vi "solar_gbl Read Config (Override).vi"(8 "error in (no error)":errorcluster, 9 "Default Targets (name,vi)":string[][](array[string]), 10 "Name in":string, 11 "SOLAR in":T1) -> (0 "error out":errorcluster, 1 "Targets (name,vi)":string[][](array[string]), 2 "Name out":string, 3 "SOLAR out":T1)   [LabVIEW 2018]
doc: "This loads the application setup override keys in the solar.ini configuration file. SOLAR uses the default application settings, to override add the key to override in the 'AppSetups' section.\nExample:\n[solar]\nAppSetups = \"Board,Box\"\nTitle = \"My Default App\"\n\n[Board]\nTitle = \"My Board App\""
uses:
  solar_ctl SOLAR Global.ctl
  solar_ctl Target Global.ctl
  voyager/solar_voy_ctl Voyager Refnum.ctl
  qtimer/solar_qtimer_ctl Refnum.ctl
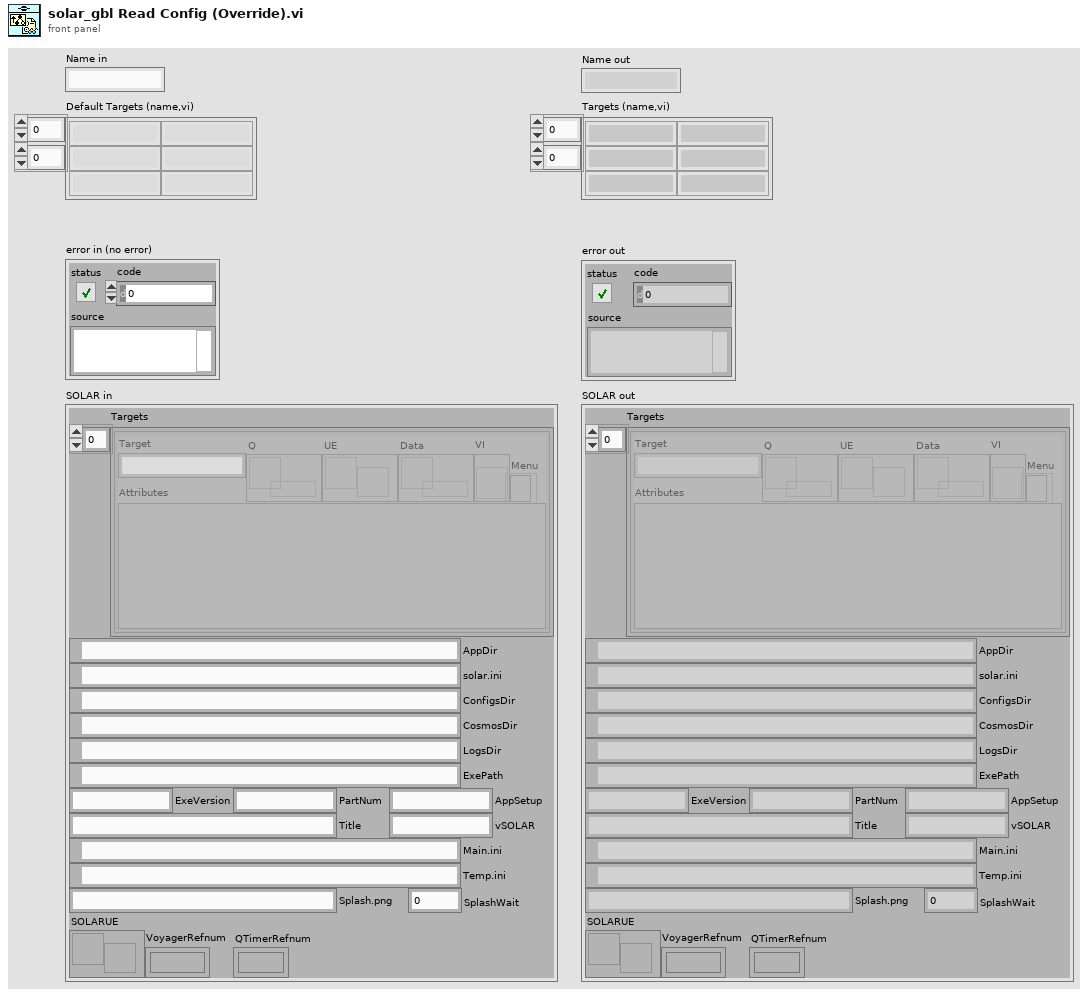
[diagram p1: front panel]
types:
  T1 = typedef "solar_ctl SOLAR Global.ctl" = cluster{"Targets":T2[], "AppDir":path, "solar.ini":path, "ConfigsDir":path, "CosmosDir":path, "LogsDir":path, "ExePath":path, "ExeVersion":string, "PartNum":string, "AppSetup":string, "Title":string, "Main.ini":path, "Temp.ini":path, "vSOLAR":string, "Splash.png":string, "SplashWait":i32, "SOLARUE":refnum<user-event>, "VoyagerRefnum":T3, "QTimerRefnum":T4}
  T2 = typedef "solar_ctl Target Global.ctl" = cluster{"Target":string, "Q":refnum<queue>, "UE":refnum<user-event>, "VI":refnum<vi>, "Menu":refnum<k9>, "Data":refnum<data-value>, "Attributes":variant}
  T3 = typedef "solar_voy_ctl Voyager Refnum.ctl" = refnum<k1>
  T4 = typedef "solar_qtimer_ctl Refnum.ctl" = refnum<k1>
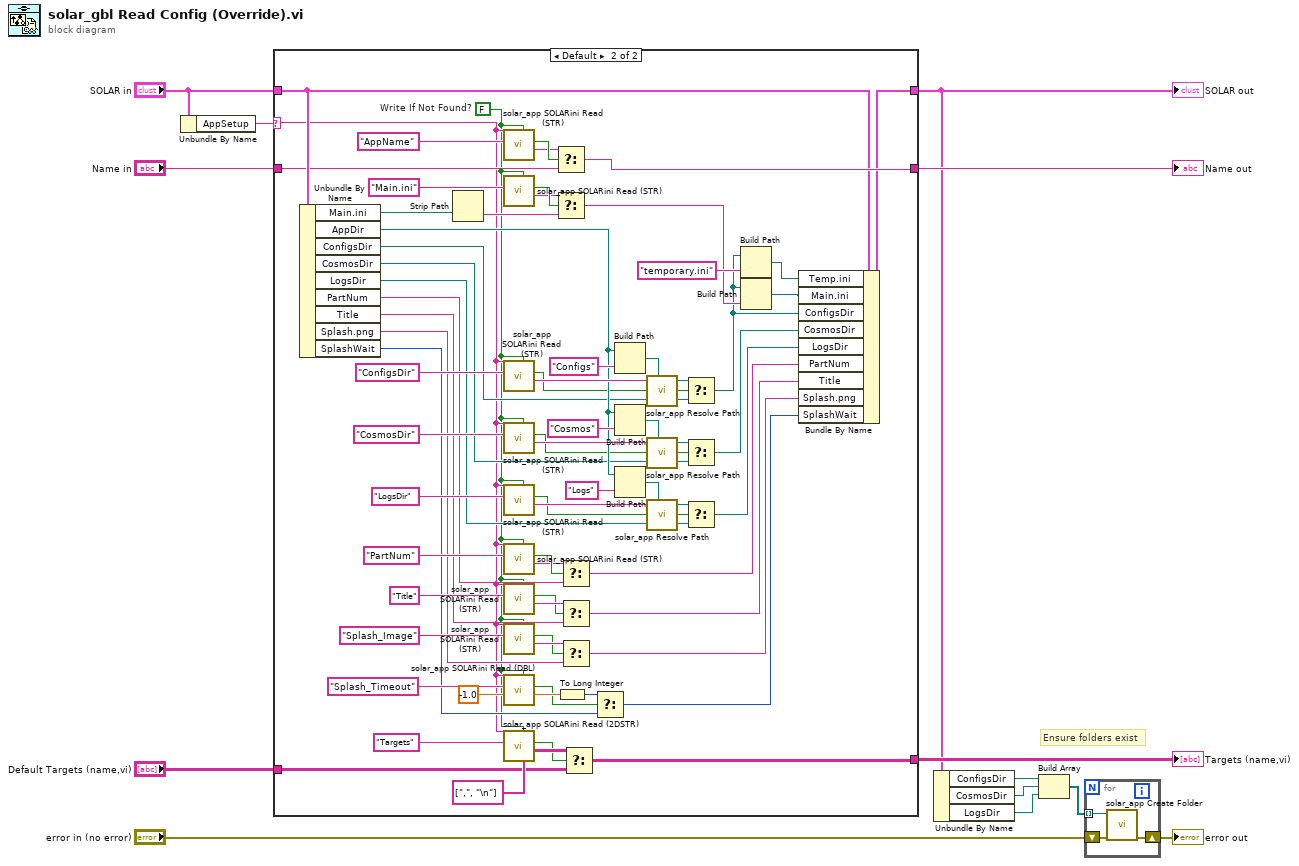
[diagram p0: block diagram]
diagram:
  # "Ensure folders exist"
  n1 = Unbundle By Name("SOLAR in") -> ("AppSetup"=w9:string)
  n2 = case shown="Default" w9 {
    selector: w9 -> [_ w18]
    tunnel: "Name in" -> [w15 w60]
    tunnel: [w15 w75] -> w12
    tunnel: [w16 w64] -> w1
    tunnel: [w14 w23] -> w11
    tunnel: "SOLAR in" -> [w16 w63]
    tunnel: "Default Targets (name,vi)" -> [w14 w24]
    frame "" {
      # "Use default configuration settings"
    }
    frame Default {
      w17 = FALSE  # Write If Not Found?
      n3 = Unbundle By Name(w63) -> ("Main.ini"=w58:path, "AppDir"=w53:path, "ConfigsDir"=w49:path, "CosmosDir"=w46:path, "LogsDir"=w40:path, "PartNum"=w37:string, "Title"=w33:string, "Splash.png"=w22:string, "SplashWait"=w20:i32)
      n4 = Strip Path(path=w58) -> (name=w57:string)  [unwired: 1 out]
      n5 = call "solar_app SOLARini Read (STR).vi"("Write If Not Found? (T)"=w17, "Section (\"\"=solar)"=w18, "Key"="AppName") -> ("Value (STR) out"=w61:string, "Found?"=w62:bool)  [unwired: 7 in]
      n6 = call "solar_app SOLARini Read (STR).vi"("Write If Not Found? (T)"=w17, "Key"="Main.ini") -> ("Value (STR) out"=w56:string, "Found?"=w59:bool)  [unwired: 8 in]
      n7 = call "solar_app SOLARini Read (STR).vi"("Write If Not Found? (T)"=w17, "Section (\"\"=solar)"=w18, "Key"="ConfigsDir") -> ("Value (STR) out"=w76:string, "Found?"=w51:bool)  [unwired: 7 in]
      n8 = call "solar_app SOLARini Read (STR).vi"("Write If Not Found? (T)"=w17, "Section (\"\"=solar)"=w18, "Key"="CosmosDir") -> ("Value (STR) out"=w78:string, "Found?"=w47:bool)  [unwired: 7 in]
      n9 = call "solar_app SOLARini Read (STR).vi"("Write If Not Found? (T)"=w17, "Section (\"\"=solar)"=w18, "Key"="LogsDir") -> ("Value (STR) out"=w81:string, "Found?"=w41:bool)  [unwired: 7 in]
      n10 = call "solar_app SOLARini Read (STR).vi"("Write If Not Found? (T)"=w17, "Section (\"\"=solar)"=w18, "Key"="PartNum") -> ("Value (STR) out"=w38:string, "Found?"=w39:bool)  [unwired: 7 in]
      n11 = call "solar_app SOLARini Read (STR).vi"("Write If Not Found? (T)"=w17, "Section (\"\"=solar)"=w18, "Key"="Title") -> ("Value (STR) out"=w35:string, "Found?"=w34:bool)  [unwired: 7 in]
      n12 = call "solar_app SOLARini Read (STR).vi"("Write If Not Found? (T)"=w17, "Section (\"\"=solar)"=w18, "Key"="Splash_Image") -> ("Value (STR) out"=w31:string, "Found?"=w28:bool)  [unwired: 7 in]
      n13 = call "solar_app SOLARini Read (DBL).vi"("Write If Not Found? (T)"=w17, "Section (\"\"=solar)"=w18, "Default Value (DBL)"=-1.0, "Key"="Splash_Timeout") -> ("Value (DBL) out"=w86:dbl, "Found?"=w29:bool)  [unwired: 6 in]
      n14 = call "solar_app SOLARini Read (2DSTR).vi"("Delimiters (1D,2D)"=string[] [",", "\n"], "Write If Not Found? (T)"=w17, "Section (\"\"=solar)"=w18, "Key"="Targets") -> ("Value (STR) out"=w26:string[][], "Found?"=w25:bool)  [unwired: 6 in]
      n15 = Select(t=w61, s=w62, f=w60) -> (s? t:f=w75:string)
      n16 = Select(t=w56, s=w59, f=w57) -> (s? t:f=w82:string)
      n17 = To Long Integer(number=w86) -> (32bit integer=w30:i32)
      n18 = Select(t=w38, s=w39, f=w37) -> (s? t:f=w36:string)
      n19 = Select(t=w35, s=w34, f=w33) -> (s? t:f=w32:string)
      n20 = Select(t=w31, s=w28, f=w22) -> (s? t:f=w21:string)
      n21 = Select(t=w26, s=w25, f=w24) -> (s? t:f=w23:string[][])
      n22 = Select(t=w30, s=w29, f=w20) -> (s? t:f=w19:i32)
      n23 = Build Path(base path=w53, name or relative path="Configs") -> (appended path=w52:path)
      n24 = Build Path(base path=w53, name or relative path="Cosmos") -> (appended path=w54:path)
      n25 = Build Path(base path=w53, name or relative path="Logs") -> (appended path=w79:path)
      n26 = call "solar_app Resolve Path.vi"("Path to Resolve (\"\"=default Path)"=w76, "default Path"=w52) -> ("Resolved Path"=w50:path)  [unwired: 6 in, 1 out]
      n27 = call "solar_app Resolve Path.vi"("Path to Resolve (\"\"=default Path)"=w78, "default Path"=w54) -> ("Resolved Path"=w48:path)  [unwired: 6 in, 1 out]
      n28 = call "solar_app Resolve Path.vi"("Path to Resolve (\"\"=default Path)"=w81, "default Path"=w79) -> ("Resolved Path"=w43:path)  [unwired: 6 in, 1 out]
      n29 = Select(t=w50, s=w51, f=w49) -> (s? t:f=w45:path)
      n30 = Select(t=w48, s=w47, f=w46) -> (s? t:f=w44:path)
      n31 = Select(t=w43, s=w41, f=w40) -> (s? t:f=w42:path)
      n32 = Build Path(base path=w45, name or relative path="temporary.ini") -> (appended path=w87:path)
      n33 = Build Path(base path=w45, name or relative path=w82) -> (appended path=w83:path)
      n34 = Bundle By Name(cluster=w63, "Temp.ini"=w87, "Main.ini"=w83, "ConfigsDir"=w45, "CosmosDir"=w44, "LogsDir"=w42, "PartNum"=w36, "Title"=w32, "Splash.png"=w21, "SplashWait"=w19) -> (w64:T1)
    }
  }
  "Name out" <- w12
  "SOLAR out" <- w1
  "Targets (name,vi)" <- w11
  n35 = Unbundle By Name(w1) -> ("ConfigsDir"=w7:path, "CosmosDir"=w6:path, "LogsDir"=w5:path)
  n36 = Build Array(w7, w6, w5) -> (w4:path[])
  n37 = for {
    shift-right: [w89] -> w2
    shift-left: "error in (no error)" -> [w90]
    tunnel: w4 -> [w88] mode=indexing
    n38 = call "solar_app Create Folder.vi"("error in (no error)"=w90, "Directory"=w88) -> ("error out"=w89:errorcluster)  [unwired: 8 in, 1 out]
  }
  "error out" <- w2
